vi "Test Position Control.vi"() -> ()   [LabVIEW 2013]
doc: "This VI tests position control of the translation table using the specified axis."
uses:
  Controls/table_axis_enum.ctl
  Controls/PWM_data_cluster.ctl
  Controls/PWM_state_enum.ctl
  <vilib>/DAQmx/write.llb/DAQmx Write (Digital Bool 1Line 1Point).vi
  <vilib>/DAQmx/write.llb/DAQmx Write (Digital 1D Bool NChan 1Samp 1Line).vi
  <vilib>/DAQmx/miscellaneous.llb/DAQmx Fill In Error Info.vi
  <vilib>/addons/control/pid/pid.llb/PID (DBL).vi
  <vilib>/addons/control/pid/NI_PID_pid.lvlib
panel:
  in  "Axis Enum":T1=enum."Z-axis"
  in  "Stop":bool
  in  "PID gains":T2={"proportional gain (Kc)"=45.0, "integral time (Ti, min)"=0.05, "derivative time (Td, min)"=0.0} {"derivative time (Td, min)" format="%.3f"; "integral time (Ti, min)" format="%.3f"; "proportional gain (Kc)" format="%.3f"}
  out "History":cluster{"Axis Inches":dbl, "output":dbl}(graph) caption="Position History"
  in  "Move Axis":bool
  out "Position (in)":dbl
  in  "Command (in)":dbl
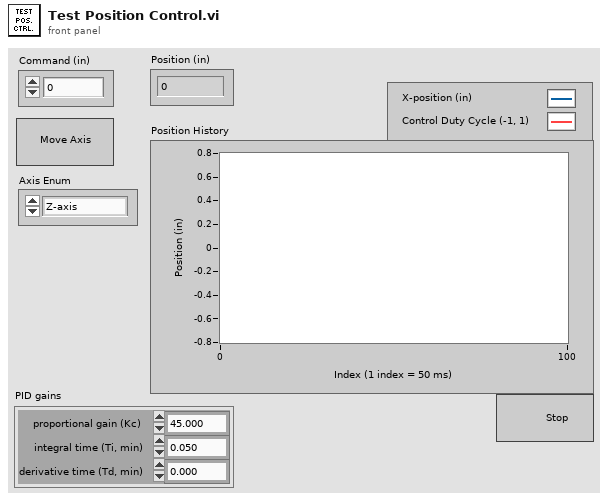
[diagram p1: front panel]
types:
  T1 = typedef "table_axis_enum.ctl" = enum16{"X-axis", "Y-axis", "Z-axis", "W-axis"}
  T2 = cluster{"proportional gain (Kc)":dbl, "integral time (Ti, min)":dbl, "derivative time (Td, min)":dbl}
  T3 = typedef "PWM_data_cluster.ctl" = cluster{"frequency":dbl, "Duty Cycle (%)":dbl, "Axis Enum":T1, "Function Enum":T4}
  T4 = typedef "PWM_state_enum.ctl" = enum16{"Initialize", "SetAxisSpeed", "StopAxis", "StopAll", "Shutdown"}
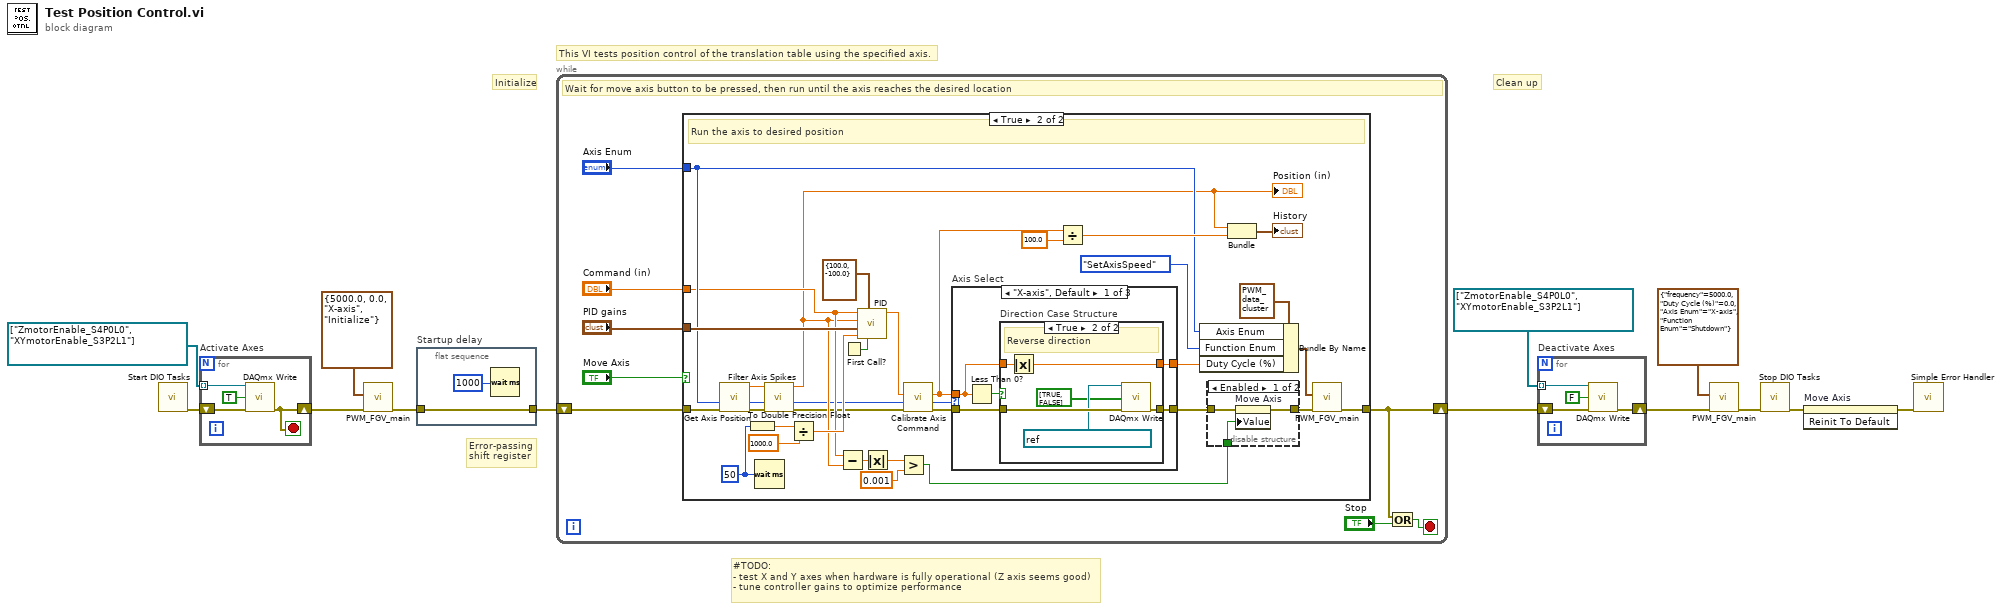
[diagram p0: block diagram]
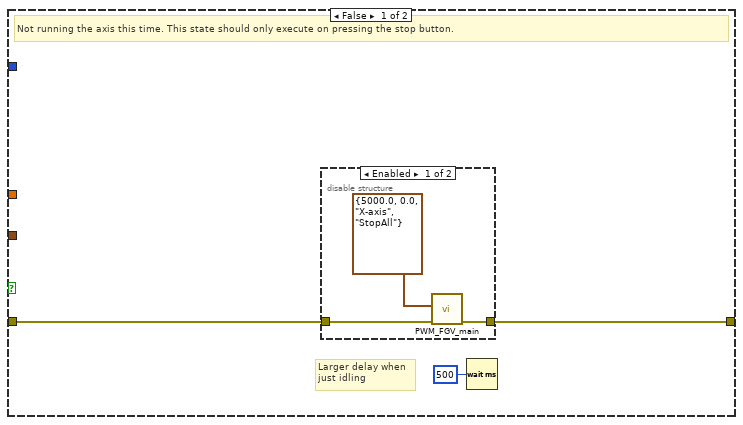
[diagram p2: hidden frame]
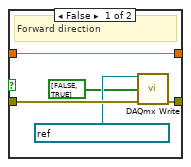
[diagram p5: hidden frame]
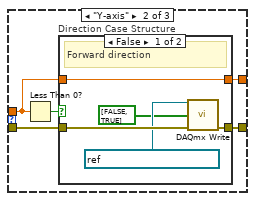
[diagram p6: hidden frame]
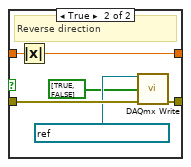
[diagram p7: hidden frame]
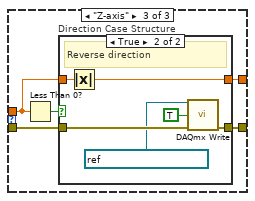
[diagram p8: hidden frame]
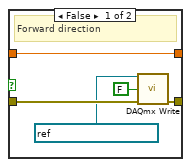
[diagram p9: hidden frame]
diagram:
  # "#TODO:\n- test X and Y axes when hardware is fully operational (Z axis seems good)\n- tune controller gains to optimize performance"
  # "Error-passing\nshift register"
  # "Clean up"
  # "Initialize"
  # "This VI tests position control of the translation table using the specified axis."
  n1 = call "Start DIO Tasks.vi"() -> ("error out"=w6:errorcluster)  [unwired: 11 in]
  n2 = for "Activate Axes" {
    shift-right: [w14] -> w5
    shift-left: w6 -> [w16]
    tunnel: refnum<k21>[] ["ZmotorEnable_S4P0L0", "XYmotorEnable_S3P2L1"] -> [w15] mode=indexing
    stop <- w14 stop-if-true
    n3 = call-poly <vilib>:"DAQmx Write.vi"("task/channels in"=w15, "data"=TRUE, "error in"=w16) -> ("error out"=w14:errorcluster)  [unwired: 10 in, 2 out]
  }
  n4 = call "PWM_FGV_main.vi"("Error In"=w5, "PWM FGV Data"=T3 {"frequency"=5000.0, "Duty Cycle (%)"=0.0, "Axis Enum"=enum."X-axis", "Function Enum"=enum."Initialize"}) -> ("Error Out"=w8:errorcluster)  [unwired: 9 in]
  n5 = flat-sequence "Startup delay" {
    tunnel: w8 -> [w19]
    tunnel: [w19] -> w7
    frame #0 {
      n6 = Wait (ms)(milliseconds to wait=u32 1000) -> ()  [unwired: 1 out]
    }
  }
  n7 = while {
    shift-right: [w21] -> w3
    shift-left: w7 -> [w27]
    stop <- w22 stop-if-true
    # "Wait for move axis button to be pressed, then run until the axis reaches the desired location"
    n8 = case shown="True" "Move Axis" {
      tunnel: w27 -> [w29 w68]
      tunnel: [w30 w67] -> w21
      tunnel: "Command (in)" -> [_ w47]
      tunnel: "PID gains" -> [_ w66]
      tunnel: "Axis Enum" -> [_ w50]
      frame False {
        # "Larger delay when\njust idling"
        # "Not running the axis this time. This state should only execute on pressing the stop button."
        n9 = disable-structure shown="Enabled" {
          disable-tunnel: [w33 w34] -> w30
          disable-tunnel: w29 -> [w32 w34]
          frame Enabled {
            n10 = call "PWM_FGV_main.vi"("Error In"=w32, "PWM FGV Data"=T3 {"frequency"=5000.0, "Duty Cycle (%)"=0.0, "Axis Enum"=enum."X-axis", "Function Enum"=enum."StopAll"}) -> ("Error Out"=w33:errorcluster)  [unwired: 9 in]
          }
          frame Disabled {
          }
        }
        n11 = Wait (ms)(milliseconds to wait=u32 500) -> ()  [unwired: 1 out]
      }
      frame True {
        w65 = u32 50 ("milliseconds to wait")
        # "Run the axis to desired position"
        n12 = call "Get Axis Position.vi"("Error In"=w68, "Axis Enum"=w50) -> ("Error Out"=w40:errorcluster, "Axis Enum Out"=w37:T1, "Axis Inches"=w39:dbl)  [unwired: 6 in, 1 out]
        n13 = To Double Precision Float(number=w65) -> (double precision float=w64:dbl)
        n14 = Wait (ms)(milliseconds to wait=w65) -> ()  [unwired: 1 out]
        n15 = call "Filter Axis Spikes.vi"("Error In"=w40, "Axis Enum"=w37, "Current Reading"=w39) -> ("Error Out"=w35:errorcluster, "Axis Enum out"=w36:T1, "Filtered Reading"=w38:dbl)  [unwired: 5 in, 1 out]
        "Position (in)" <- w38
        n16 = Divide(x=w64, y=1000.0) -> (x/y=w61:dbl)
        n17 = Subtract(x=w47, y=w38) -> (x-y=w46:dbl)
        n18 = First Call?() -> (First Call?: T/F=w62:bool)
        n19 = call-poly <vilib>:"PID.vi"("reinitialize? (F)"=w62, "output range"=cluster{"output high":dbl, "output low":dbl} {"output high"=100.0, "output low"=-100.0}, "dt (s)"=w61, "PID gains"=w66, "process variable"=w38, "setpoint"=w47) -> ("output"=w51:dbl)  [unwired: 4 in, 1 out]
        n20 = Absolute Value(x=w46) -> (abs(x)=w45:dbl)
        n21 = Greater?(x=w45, y=0.001) -> (0:w41:bool)
        n22 = call "Calibrate Axis Command.vi"("Error In"=w35, "Axis Enum"=w36, "Duty Cycle (%)"=w51) -> ("Error Out"=w52:errorcluster, "Axis Enum out"=w48:T1, "Calib. Duty Cycle"=w49:dbl)  [unwired: 6 in]
        n23 = case "Axis Select" shown="\"X-axis\", Default" w48 {
          tunnel: [w76 w92 w108] -> w43
          tunnel: [w75 w91 w107] -> w53
          tunnel: w52 -> [w74 w90 w106]
          tunnel: w49 -> [w73 w89 w105]
          frame "X-axis", Default {
            n24 = Less Than 0?(x=w73) -> (x < 0?=w77:bool)
            n25 = case "Direction Case Structure" shown="True" w77 {
              tunnel: w74 -> [w80 w85]
              tunnel: [w81 w86] -> w76
              tunnel: w73 -> [w82 w88]
              tunnel: [w82 w87] -> w75
              frame False {
                # "Forward direction"
                n26 = call-poly <vilib>:"DAQmx Write.vi"("task/channels in"=refnum<k21> "Xdirection_S3P2L2-3", "data"=bool[] [FALSE, TRUE], "error in"=w80) -> ("error out"=w81:errorcluster)  [unwired: 10 in, 2 out]
              }
              frame True {
                # "Reverse direction"
                n27 = Absolute Value(x=w88) -> (abs(x)=w87:dbl)
                n28 = call-poly <vilib>:"DAQmx Write.vi"("task/channels in"=refnum<k21> "Xdirection_S3P2L2-3", "data"=bool[] [TRUE, FALSE], "error in"=w85) -> ("error out"=w86:errorcluster)  [unwired: 10 in, 2 out]
              }
            }
          }
          frame "Y-axis" {
            n29 = Less Than 0?(x=w89) -> (x < 0?=w93:bool)
            n30 = case "Direction Case Structure" shown="False" w93 {
              tunnel: w90 -> [w96 w101]
              tunnel: [w97 w102] -> w92
              tunnel: w89 -> [w98 w104]
              tunnel: [w98 w103] -> w91
              frame False {
                # "Forward direction"
                n31 = call-poly <vilib>:"DAQmx Write.vi"("task/channels in"=refnum<k21> "Ydirection_S3P2L6-7", "data"=bool[] [FALSE, TRUE], "error in"=w96) -> ("error out"=w97:errorcluster)  [unwired: 10 in, 2 out]
              }
              frame True {
                # "Reverse direction"
                n32 = Absolute Value(x=w104) -> (abs(x)=w103:dbl)
                n33 = call-poly <vilib>:"DAQmx Write.vi"("task/channels in"=refnum<k21> "Ydirection_S3P2L6-7", "data"=bool[] [TRUE, FALSE], "error in"=w101) -> ("error out"=w102:errorcluster)  [unwired: 10 in, 2 out]
              }
            }
          }
          frame "Z-axis" {
            n34 = Less Than 0?(x=w105) -> (x < 0?=w109:bool)
            n35 = case "Direction Case Structure" shown="True" w109 {
              tunnel: w106 -> [w112 w118]
              tunnel: [w113 w119] -> w108
              tunnel: w105 -> [w114 w120]
              tunnel: [w114 w115] -> w107
              frame False {
                # "Forward direction"
                n36 = call-poly <vilib>:"DAQmx Write.vi"("task/channels in"=refnum<k21> "Zdirection_S4P0L1", "data"=FALSE, "error in"=w112) -> ("error out"=w113:errorcluster)  [unwired: 10 in, 2 out]
              }
              frame True {
                # "Reverse direction"
                n37 = Absolute Value(x=w120) -> (abs(x)=w115:dbl)
                n38 = call-poly <vilib>:"DAQmx Write.vi"("task/channels in"=refnum<k21> "Zdirection_S4P0L1", "data"=TRUE, "error in"=w118) -> ("error out"=w119:errorcluster)  [unwired: 10 in, 2 out]
              }
            }
          }
        }
        n39 = Divide(x=w49, y=100.0) -> (x/y=w55:dbl)
        n40 = Bundle By Name(cluster=T3 {"frequency"=5000.0, "Duty Cycle (%)"=0.0, "Axis Enum"=enum."X-axis", "Function Enum"=enum."Shutdown"} ("PWM FGV Data"), "Axis Enum"=w50, "Function Enum"=PWM_state_enum."SetAxisSpeed", "Duty Cycle (%)"=w53) -> (w58:T3)
        n41 = disable-structure shown="Enabled" {
          disable-tunnel: w43 -> [w71 w72]
          disable-tunnel: [w70 w72] -> w42
          disable-tunnel: w41 -> [w69 _]
          frame Enabled {
            n42 = property on="Move Axis" class="Bool (strict)"(error in=w71, "Value"=w69) -> (error out=w70:errorcluster)  [unwired: 1 in, 1 out]
          }
          frame Disabled {
          }
        }
        n43 = Bundle("Filtered Reading"=w38, w55) -> (→"History":cluster{"Filtered Reading":dbl, dbl})  [unwired: 1 in]
        n44 = call "PWM_FGV_main.vi"("Error In"=w42, "PWM FGV Data"=w58) -> ("Error Out"=w67:errorcluster)  [unwired: 9 in]
      }
    }
    n45 = Or(x=w21, y="Stop") -> (x .or. y?=w22:bool)
  }
  n46 = for "Deactivate Axes" {
    shift-right: [w122] -> w2
    shift-left: w3 -> [w123]
    tunnel: refnum<k21>[] ["ZmotorEnable_S4P0L0", "XYmotorEnable_S3P2L1"] -> [w121] mode=indexing
    n47 = call-poly <vilib>:"DAQmx Write.vi"("task/channels in"=w121, "data"=FALSE, "error in"=w123) -> ("error out"=w122:errorcluster)  [unwired: 10 in, 2 out]
  }
  n48 = call "PWM_FGV_main.vi"("Error In"=w2, "PWM FGV Data"=T3 {"frequency"=5000.0, "Duty Cycle (%)"=0.0, "Axis Enum"=enum."X-axis", "Function Enum"=enum."Shutdown"}) -> ("Error Out"=w12:errorcluster)  [unwired: 9 in]
  n49 = call "Stop DIO Tasks.vi"("Error In"=w12) -> ("error out"=w10:errorcluster)  [unwired: 10 in]
  n50 = invoke on="Move Axis" class="Bool (strict)" method="Reinit To Default"(error in=w10) -> (error out=w9:errorcluster)  [unwired: 2 in, 2 out]
  n51 = call <vilib>:"Simple Error Handler.vi"("error in (no error)"=w9) -> ()  [unwired: 4 in, 5 out]
